vi "Read PRACH Modulation Results.vi"(0 "VISA resource name":refnum<visa-resource-name>, 5 "Instance (1)":T1=1, 7 "Result Type (Current)":i32(ring) items=["Current"=0, "Average"=1, "Standard Deviation"=3], 11 "error in (no error)":errorcluster) -> (4 "VISA resource name out":refnum<visa-resource-name>, 6 "Reliability":i32, 8 "Out Of Tolerance":i32, 10 "Results":dbl[](array[numeric]) format="%^.3e", 15 "error out":errorcluster)   [LabVIEW 2020, in "Rohde&Schwarz CMWXP NR FR1 Measurement.lvlib"]
doc: "Starts a new single shot measurement and returns the single value modulation results.\n\nAttributes:\nRSCMWXPNRFR1M_ATTR_READ_PRACH_MODULATION_CURRENT_RESULTS\nRSCMWXPNRFR1M_ATTR_READ_PRACH_MODULATION_AVERAGE_RESULTS\nRSCMWXPNRFR1M_ATTR_READ_PRACH_MODULATION_STANDARD_DEVIATION_RESULTS\n\nRemote-control commands:\nREAD:NRSub:MEAS<i>:PRACh:MODulation:CURRent?\nREAD:NRSub:MEAS<i>:PRACh:MODulation:AVERage?\nREAD:NRSub:MEAS<i>:PRACh:MODulation:SDEViation?"
uses:
  <instrlib>/Rohde&Schwarz CMWXP NR FR1 Measurement/Rohde&Schwarz CMWXP NR FR1 Measurement.lvlib
  <instrlib>/Rohde&Schwarz CMWXP NR FR1 Measurement/Private/_Instance.ctl
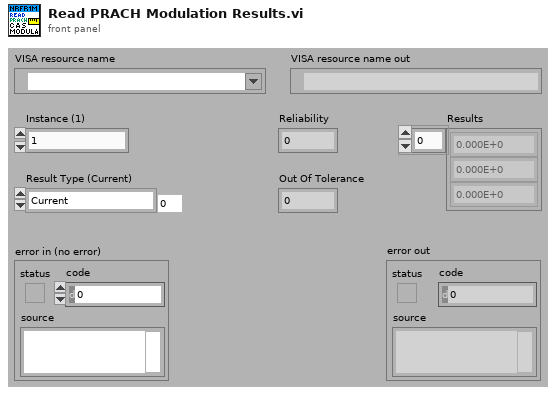
[diagram p1: front panel]
types:
  T1 = typedef "Rohde&Schwarz CMWXP NR FR1 Measurement.lvlib/_Instance.ctl" = i32
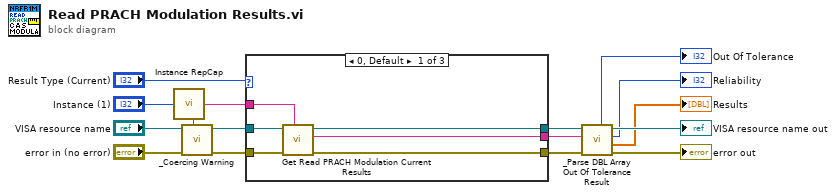
[diagram p0: block diagram]
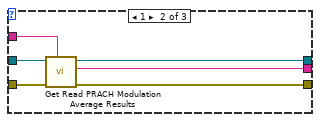
[diagram p2: hidden frame]
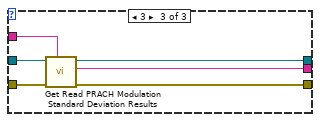
[diagram p3: hidden frame]
diagram:
  n1 = call <instrlib>:"Instance RepCap.vi"("Instance In"="Instance (1)") -> ("In Range?"=w16:bool, "RepCap Identifier Out"=w13:string)  [unwired: 1 in]
  n2 = call <instrlib>:"_Coercing Warning.vi"("In Range?"=w16, "error in (no error)"="error in (no error)", "VISA resource name"="VISA resource name") -> ("error out"=w15:errorcluster, "VISA resource name out"=w14:refnum<visa-resource-name>)  [unwired: 7 in]
  n3 = case shown="0, Default" "Result Type (Current)" {
    tunnel: w14 -> [w22 w28 w34]
    tunnel: w15 -> [w21 w27 w33]
    tunnel: w13 -> [w20 w26 w32]
    tunnel: [w19 w25 w29] -> w7
    tunnel: [w18 w24 w31] -> w6
    tunnel: [w17 w23 w30] -> w5
    frame 0, Default {
      n4 = call "Get Read PRACH Modulation Current Results"("Repeated Capabilities"=w20, "error in (no error)"=w21, "instrument handle"=w22) -> ("error out"=w19:errorcluster, "Read PRACH Modulation Current Results"=w17:string, "instrument handle out"=w18:refnum<visa-resource-name>)  [unwired: 6 in]
    }
    frame 1 {
      n5 = call "Get Read PRACH Modulation Average Results"("Repeated Capabilities"=w26, "error in (no error)"=w27, "instrument handle"=w28) -> ("error out"=w25:errorcluster, "Read PRACH Modulation Average Results"=w23:string, "instrument handle out"=w24:refnum<visa-resource-name>)  [unwired: 6 in]
    }
    frame 3 {
      n6 = call "Get Read PRACH Modulation Standard Deviation Results"("Repeated Capabilities"=w32, "error in (no error)"=w33, "instrument handle"=w34) -> ("error out"=w29:errorcluster, "Read PRACH Modulation Standard Deviation Results"=w30:string, "instrument handle out"=w31:refnum<visa-resource-name>)  [unwired: 6 in]
    }
  }
  n7 = call <instrlib>:"_Parse DBL Array Out Of Tolerance Result.vi"("error in (no error)"=w7, "Input String"=w5, "VISA resource name"=w6) -> ("error out"=→"error out":errorcluster, "Results"=→"Results":dbl[], "Reliability"=→"Reliability":i32, "VISA resource name out"=→"VISA resource name out":refnum<visa-resource-name>, "Out Of Tolerance"=→"Out Of Tolerance":i32)  [unwired: 4 in]
